vi "GdsLanguage_GOOPKernel.vi"(1 "Data in":T1, 5 "error in (no error)":errorcluster, 6 "Action":enum16{"Get", "Set"}(ring)) -> (15 "Data out":T1, 19 "error out":errorcluster)   [LabVIEW 2014]
doc: "This VIs manages objects of the AcTranslator.\n\n[GOOP 2.0.13]"
uses:
  <resource>/Framework/Providers/Open_GDS/ClassProviders/Common/GdsLanguage/private/GdsLanguage_ObjectAttributes.ctl
  <resource>/Framework/Providers/Open_GDS/ClassProviders/Common/GdsLanguage/GdsLanguage_LanguageID.ctl
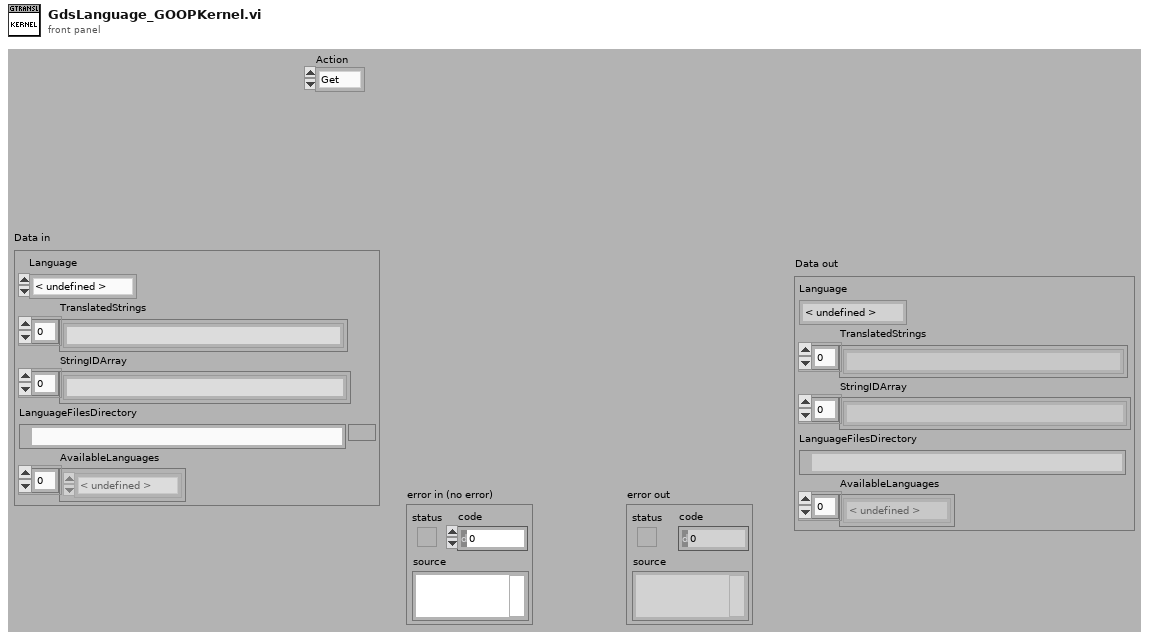
[diagram p1: front panel]
types:
  T1 = typedef "GdsLanguage_ObjectAttributes.ctl" = cluster{"Language":T2, "TranslatedStrings":string[], "StringIDArray":string[], "LanguageFilesDirectory":path, "AvailableLanguages":T2[]}
  T2 = typedef "GdsLanguage_LanguageID.ctl" = enum16{"< undefined >", "aa", "ab", "af", "am", "ar", "as", "ay", "az", "ba", "be", "bg", "bh", "bi", "bn", "bo", "br", "ca", "co", "cs", "cy", "da", "de", "dz", "el", "en", "eo", "es", "et", "eu", "fa", "fi", "fj", "fo", "fr", "fy", "ga", "gd", "gl", "gn", "gu", "gv", "ha", "he", "hi", "hr", "hu", "hy", "ia", "id", "ie", "ik", "is", "it", "iu", "ja", "jv", "ka", "kk", "kl", "km", "kn", "ko", "ks", "ku", "ky", "la", "li", "ln", "lo", "lt", "lv", "mg", "mi", "mk", "ml", "mn", "mo", "mr", "ms", "mt", "my", "na", "ne", "nl", "no", "oc", "om", "or", "pa", "pl", "ps", "pt", "qu", "rm", "rn", "ro", "ru", "rw", "sa", "sd", "sg", "sh", "si", "sk", "sl", "sm", "sn", "so", "sq", "sr", "ss", "st", "su", "sv", "sw", "ta", "te", "tg", "th", "ti", "tk", "tl", "tn", "to", "tr", "ts", "tt", "tw", "ug", "uk", "ur", "uz", "vi", "vo", "wo", "xh", "yi", "yo", "zh", "zu"}
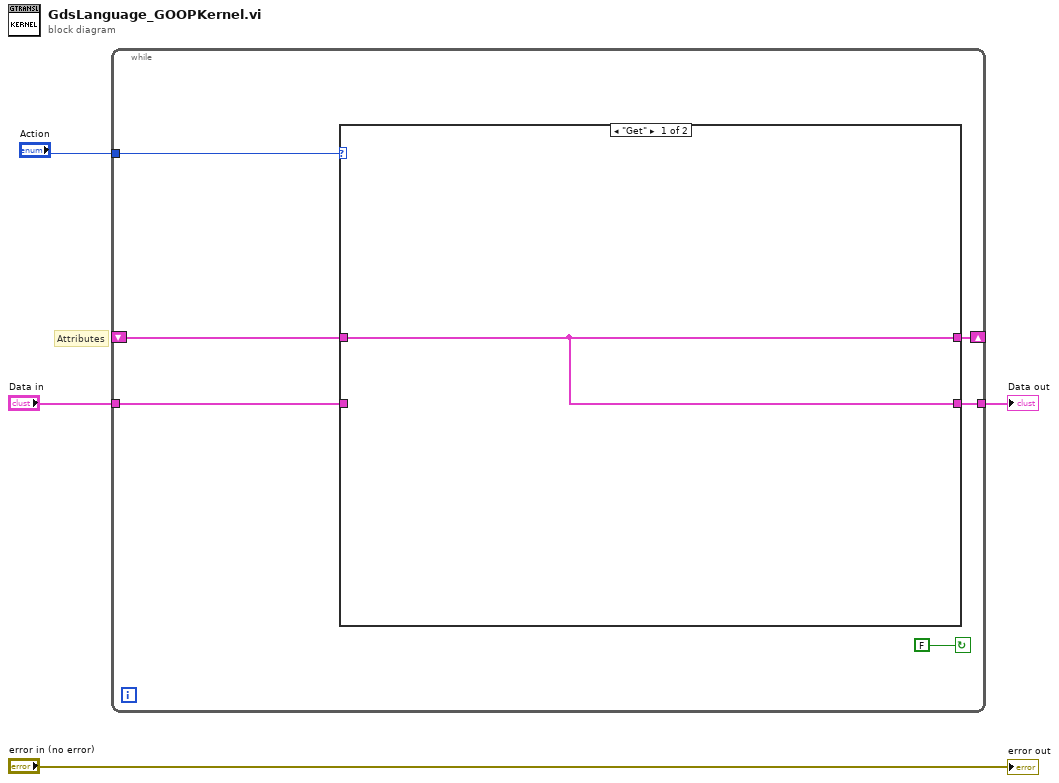
[diagram p0: block diagram]
diagram:
  # "Attributes"
  n1 = while {
    shift-left: _ -> [w8]
    shift-right: [w9] -> _
    tunnel: [w10] -> w3
    tunnel: "Data in" -> [w7]
    tunnel: "Action" -> [w5]
    stop <- FALSE continue-if-true
    n2 = case shown="\"Get\"" w5 {
      tunnel: [w11 w12] -> w10
      tunnel: [w11 w12] -> w9
      tunnel: w8 -> [w11 _]
      tunnel: w7 -> [_ w12]
      frame "Get" {
      }
      frame "Set" {
      }
    }
  }
  "Data out" <- w3
  "error out" <- "error in (no error)"
